vi "Get Actor Handles.vi"() -> (2 "Actor Handles":refnum<class "Protected Actor Handle.lvclass">[](array[class]))   [LabVIEW 2020, in "AF Debug.lvlib"]
doc: "This VI returns an array of handles for currently running actors to use in a debugging tool. Actors are wrapped in handles to limit a debugger's ability to interfere with the operation of the actors and to protect the debugger from actors stopping unexpectedly.\n\nThis VI is a wrapper for a VI of the same name in Actor Framework.lvlib. It has been provided to support tools written to use older versions of the AF Debug library. It is DEPRECATED, but functional."
uses:
  AFDebug/AF Debug.lvlib
  Actor Framework.lvlib
  Inspection API/Protected Actor Handle/Protected Actor Handle.lvclass
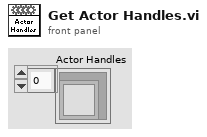
[diagram p1: front panel]
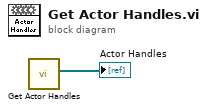
[diagram p0: block diagram]
diagram:
  n1 = call "Get Actor Handles.vi"() -> ("Actor Handles"=→"Actor Handles":refnum<class "Protected Actor Handle.lvclass">[])  [unwired: 11 in]
